vi "Streamer_Create.vi"(0 "reference in":refnum<class "Streamer.lvclass">, 2 "Stream Queues":refnum<queue>[](array[refnum]), 3 "HPS17K Ref":refnum<class "HPS-17000.lvclass">, 5 "Error In":errorcluster) -> (14 "reference out":refnum<class "Streamer.lvclass">, 19 "Error Out":errorcluster)   [LabVIEW 2023, in "Streamer.lvclass"]
uses:
  Streamer.lvclass
  <instrlib>/HPS-17000/HPS-17000.lvclass
  <vilib>/HPS-17000/MStream_grpc_CyclerMeasurement.ctl
  Streamer.lvclass/Streamer.ctl
  <vilib>/HPS-17000/NI_BC_client.lvlib
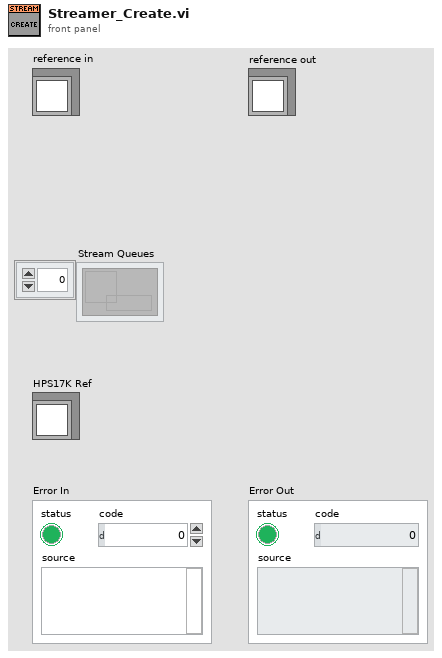
[diagram p1: front panel]
types:
  T1 = typedef "Streamer.lvclass/ObjectAttributes.ctl" = cluster{"Stream Queues":refnum<queue>[], "HPS17K Ref":refnum<class "HPS-17000.lvclass">}
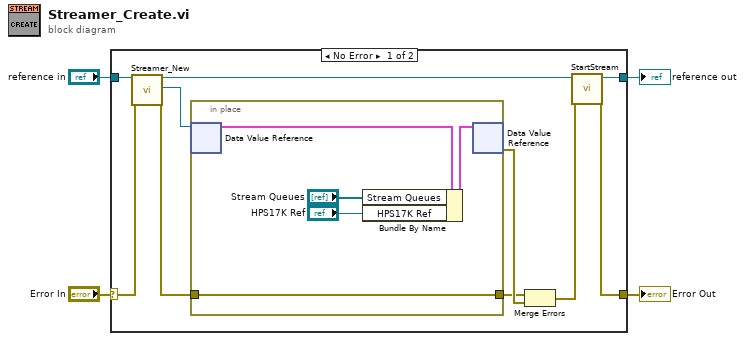
[diagram p0: block diagram]
diagram:
  n1 = case shown="No Error" "Error In" {
    selector: "Error In" -> [w13 w21]
    tunnel: [w5 w21] -> w3
    tunnel: "reference in" -> [w14 w20]
    tunnel: [w7 w20] -> w1
    frame No Error {
      n2 = call "Streamer_New.vi"("reference in"=w14, "Error In"=w13) -> ("reference out"=w8:refnum<class "Streamer.lvclass">, "DVRRefOut"=w11:refnum<data-value>, "Error Out"=w10:errorcluster)  [unwired: 14 in, 1 out]
      n3 = in-place {
        in-place-border: w10 -> [w17]
        in-place-border: [w17] -> w9
        n4 = in-place-dvr #1(w11) -> (w18:T1)  [unwired: 1 out]
        n5 = Bundle By Name(cluster=w18, "Stream Queues"="Stream Queues", "HPS17K Ref"="HPS17K Ref") -> (w19:T1)
        n6 = in-place-dvr #1(w19) -> (w12:errorcluster)  [unwired: 1 out]
      }
      n7 = Merge Errors(w9, w12) -> (w6:errorcluster)
      n8 = call "StartStream.vi"("reference in"=w8, "Error In"=w6) -> ("reference out"=w7:refnum<class "Streamer.lvclass">, "Error Out"=w5:errorcluster)  [unwired: 14 in, 2 out]
    }
    frame Error {
      # "VI-TechBaseTemplate_Simple_6x8x6"
    }
  }
  "Error Out" <- w3
  "reference out" <- w1
